vi "PathPlanner_Trajectory_WriteCSVFileStates.vi"(9 "Trajectory":T1 {"States"."TargetHolonomicRotation"."SIN" format="%13.4f"; "States"."TargetHolonomicRotation"."COS" format="%13.4f"; "States"."TargetHolonomicRotation"."VALUE" format="%13.4f"; "States"."Heading"."SIN" format="%13.4f"; "States"."Heading"."COS" format="%13.4f"; "States"."Heading"."VALUE" format="%13.4f"; "States"."PositionMeters"."Y" format="%14.3f"; "States"."PositionMeters"."X" format="%14.3f"}, 11 "Byte Steam File In":refnum<file>) -> (0 "error out":errorcluster, 3 "Byte Steam File Out":refnum<file>)   [LabVIEW 2019]
doc: "Write trajectory states to a file. This is an internal routine\n\nParameters:\n - ByteStreamIn - File stream\n - Trajectory - Data structure containing trajectory\n\nReturns:\n - ByteStreamOut - File stream\n - Error out - returned error cluster"
uses:
  TypeDef/PathPlannerTrajectory.ctl
  TypeDef/PathPlannerTrajectoryState.ctl
  <vilib>/Rock Robotics/WPI/ThirdParty/JAS_Junk/TrajLib/TypeDef/TRANSLATION2D.ctl
  <vilib>/Rock Robotics/WPI/ThirdParty/JAS_Junk/TrajLib/TypeDef/ROTATION2D.ctl
  TypeDef/PathPlannerPathConstraints.ctl
  <vilib>/Rock Robotics/WPI/ThirdParty/JAS_Junk/TrajLib/Trajectory_Library.lvlib
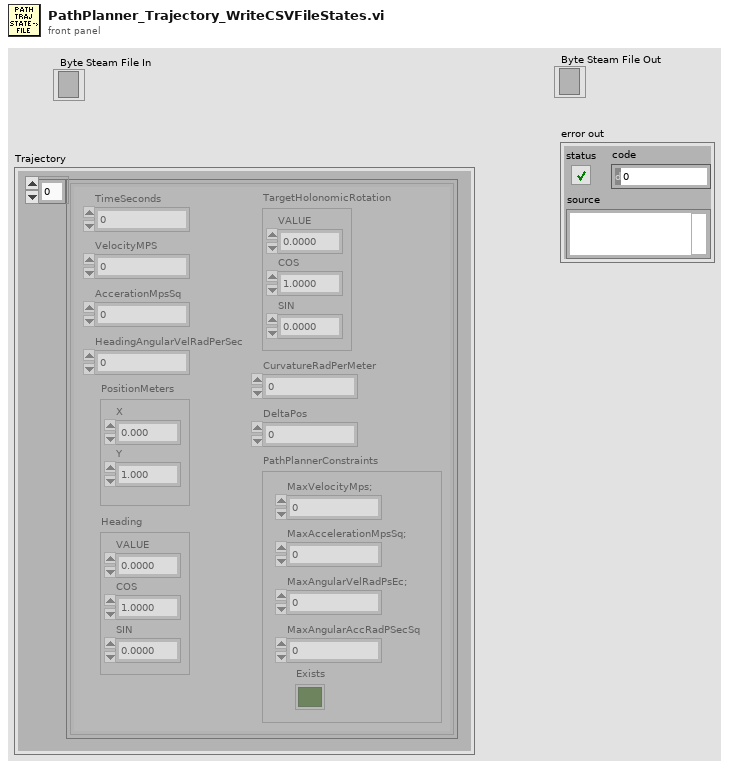
[diagram p1: front panel]
types:
  T1 = typedef "PathPlannerTrajectory.ctl" = cluster{"States":T2[]}
  T2 = typedef "PathPlannerTrajectoryState.ctl" = cluster{"TimeSeconds":dbl, "VelocityMPS":dbl, "AccerationMpsSq":dbl, "HeadingAngularVelRadPerSec":dbl, "PositionMeters":T3, "Heading":T4, "TargetHolonomicRotation":T4, "CurvatureRadPerMeter":dbl, "PathPlannerConstraints":T5, "DeltaPos":dbl}
  T3 = typedef "Trajectory_Library.lvlib/TRANSLATION2D.ctl" = cluster{"X":dbl, "Y":dbl}
  T4 = typedef "Trajectory_Library.lvlib/ROTATION2D.ctl" = cluster{"VALUE":dbl, "COS":dbl, "SIN":dbl}
  T5 = typedef "PathPlannerPathConstraints.ctl" = cluster{"MaxVelocityMps;":dbl, "MaxAccelerationMpsSq;":dbl, "MaxAngularVelRadPsEc;":dbl, "MaxAngularAccRadPSecSq":dbl, "Exists":bool}
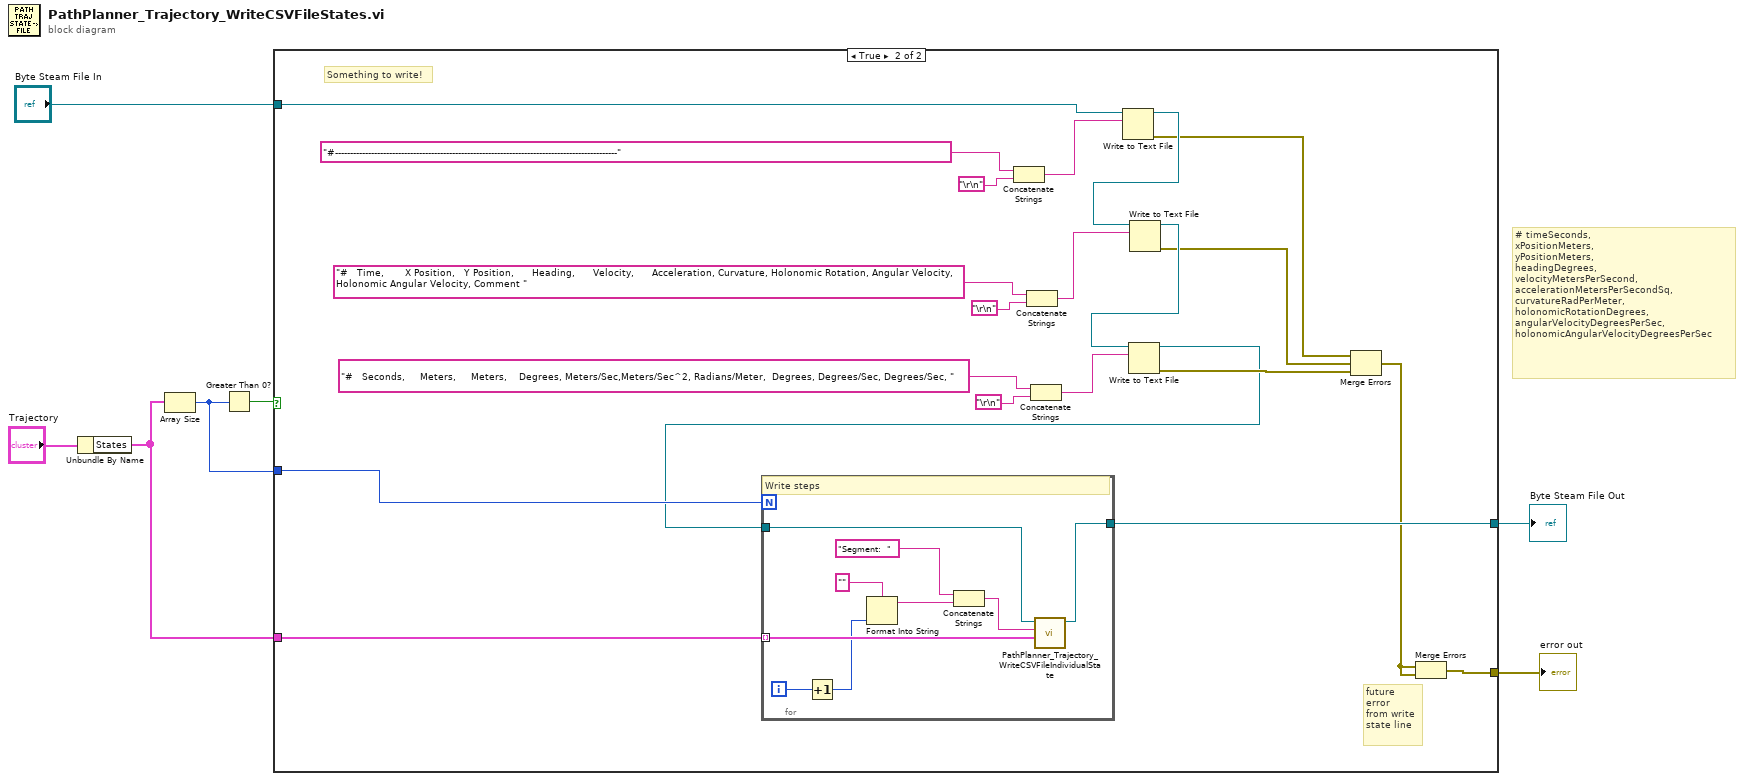
[diagram p0: block diagram]
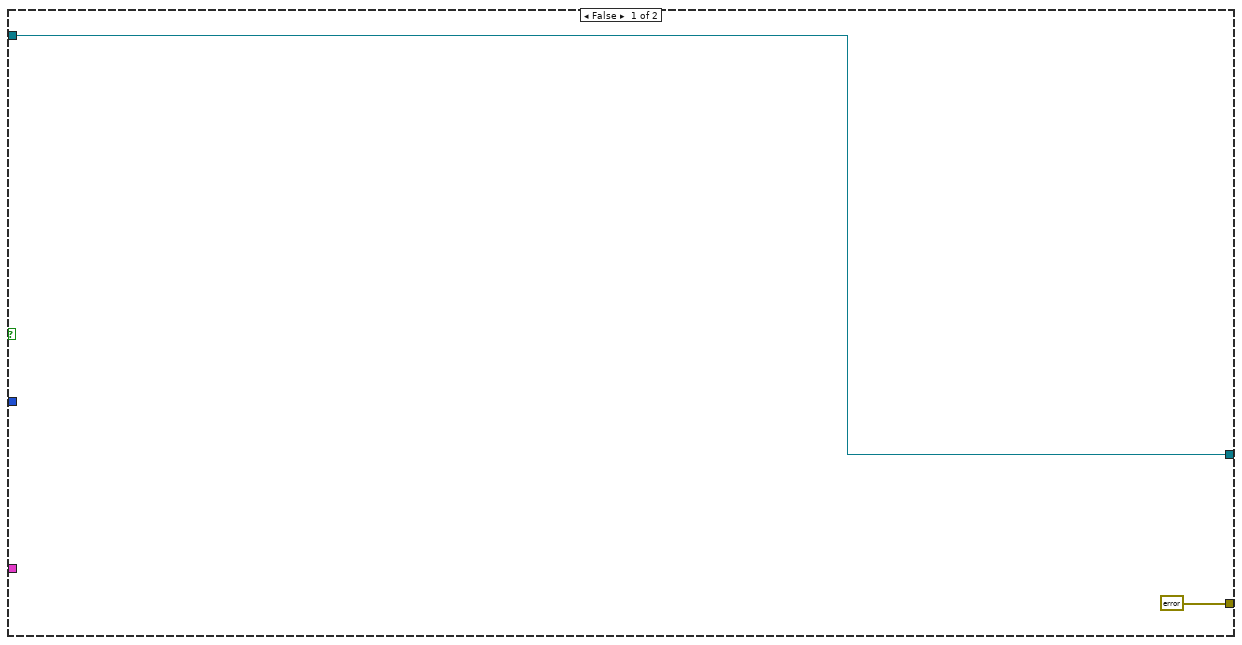
[diagram p2: hidden frame]
diagram:
  # "# timeSeconds, \nxPositionMeters, \nyPositionMeters, \nheadingDegrees, \nvelocityMetersPerSecond, \naccelerationMetersPerSecondSq, \ncurvatureRadPerMeter, \nholonomicRotationDegrees, \nangularVelocityDegreesPerSec, \nholonomicAngularVelocityDegreesPerSec"
  n1 = Unbundle By Name("Trajectory") -> ("States"=w2:T2[])
  n2 = Array Size(array=w2) -> (size(s)=w3:i32)
  n3 = Greater Than 0?(x=w3) -> (x > 0?=w6:bool)
  n4 = case shown="True" w6 {
    tunnel: [w9 w12] -> w7
    tunnel: w3 -> [_ w14]
    tunnel: "Byte Steam File In" -> [w9 w21]
    tunnel: [errorcluster {"status"=FALSE, "code"=0, "source"=""} ("error out") w15] -> w4
    tunnel: w2 -> [_ w11]
    frame False {
    }
    frame True {
      # "future\nerror\nfrom write\nstate line"
      # "Something to write!"
      n5 = Concatenate Strings("#----------------------------------------------------------------------------------------------" ("string"), "\r\n") -> (w22:string)
      n6 = Concatenate Strings("#   Time,       X Position,   Y Position,      Heading,      Velocity,      Acceleration, Curvature, Holonomic Rotation, Angular Velocity, Holonomic Angular Velocity, Comment " ("string"), "\r\n") -> (w28:string)
      n7 = Concatenate Strings("#   Seconds,     Meters,     Meters,    Degrees, Meters/Sec,Meters/Sec^2, Radians/Meter,  Degrees, Degrees/Sec, Degrees/Sec, " ("string"), "\r\n") -> (w23:string)
      n8 = Write to Text File(file (use dialog)=w21, text=w22) -> (refnum out=w20:refnum<file>, error out=w18:errorcluster)  [unwired: 2 in, 1 out]
      n9 = Write to Text File(file (use dialog)=w20, text=w28) -> (refnum out=w19:refnum<file>, error out=w17:errorcluster)  [unwired: 2 in, 1 out]
      n10 = Write to Text File(file (use dialog)=w19, text=w23) -> (refnum out=w13:refnum<file>, error out=w16:errorcluster)  [unwired: 2 in, 1 out]
      n11 = for {
        N: w14 -> [_]
        tunnel: w11 -> [w33] mode=indexing
        tunnel: [w39] -> w12
        tunnel: w13 -> [w38]
        i -> [w31]
        # "Write steps"
        n12 = Increment(x=w31) -> (x+1=w32:i32)
        n13 = Format Into String(format string="", w32) -> (resulting string=w36:string)  [unwired: 2 in, 1 out]
        n14 = Concatenate Strings("Segment:  " ("string"), w36) -> (w34:string)
        n15 = call "PathPlanner_Trajectory_WriteCSVFileIndividualState.vi"("PathPlannerState"=w33, "Comment"=w34, "Byte Stream File in"=w38) -> ("Byte Stream File out"=w39:refnum<file>)  [unwired: 8 in]
      }
      n16 = Merge Errors(w18, w17, w16) -> (w10:errorcluster)
      n17 = Merge Errors(w10, w10) -> (w15:errorcluster)
    }
  }
  "error out" <- w4
  "Byte Steam File Out" <- w7
